vi "RDB Create Objects.vi"(8 "error in":errorcluster, 11 "Compiled.Settings":T5={"Name"="", "RDB Data Receive "=[], "RDB Data Sent"=[], "vclient"=path "", "Network Settings"={"IP adress"="127.0.0.1", "RDB"={"Protocol"=enum."UDP", "Tx Port"=48270, "Rx Port"=10, "Buffer Size"=204800, "Timeout"=10}, "SCP"={"Protocol"=enum."TCP", "Tx Port"=48191, "Rx Port"=48191, "Buffer Size"=204800, "Timeout"=10}}, "SensorInfos"=[], "mmanager"=path "", "Scenario Paths"=[], "Custom SCP Commands"=[]}) -> (0 "error out":errorcluster, 3 "RDB References":T1 {"RDB Send Reference"."RDB Data"."payload" format="%x"; "RDB Send Reference"."RDB Data"."timestamp" format="%<%.7X\n%x>T"; "RDB Send Reference"."RDB Data"."type" items=["FlexRay Data"=32, "FlexRay Null"=33, "FlexRay Symbol"=34, "Log Trigger"=225, "Start Trigger"=226]; "RDB Send Reference"."RDB Data"."cycle count" max=63 step=1; "RDB Receive Reference"."RDB Data"."payload" format="%x"; "RDB Receive Reference"."RDB Data"."timestamp" format="%<%.7X\n%x>T"; "RDB Receive Reference"."RDB Data"."type" items=["FlexRay Data"=32, "FlexRay Null"=33, "FlexRay Symbol"=34, "Log Trigger"=225, "Start Trigger"=226]; "RDB Receive Reference"."RDB Data"."cycle count" max=63 step=1})   [LabVIEW 2023, in "RDB.lvlib"]
uses:
  RDB.lvlib
  Shared/Compiled.Settings.ctl
  System Explorer/RDB Data.ctl
  RDB Object.ctl
  RDB Player Object.ctl
  Shared/Network Settings.ctl
  Shared/Protocol.ctl
  Shared/SensorInfos.ctl
  Shared/SensorInfo.ctl
  Shared/Sensor Name.ctl
  MM/MM Data.ctl
  MM/MM Objects.ctl
  MM/MM Object.ctl
  RDB References.ctl
  RDB Reference.ctl
  <vilib>/xnet/xnet.llb/XNET Frame FlexRay.ctl
  <vilib>/xnet/xnet.llb/XNET Frame Type FlexRay.ctl
  <vilib>/xnet/xnet.llb/XNET String To IO Name (Signal).vi
  <vilib>/xnet/xnet.llb/XNET Create Session (Conversion).vi
  <resource>/objmgr/xnet.rc
  Shared/Vires VTD Shared.lvlib
  MM/MM.lvlib
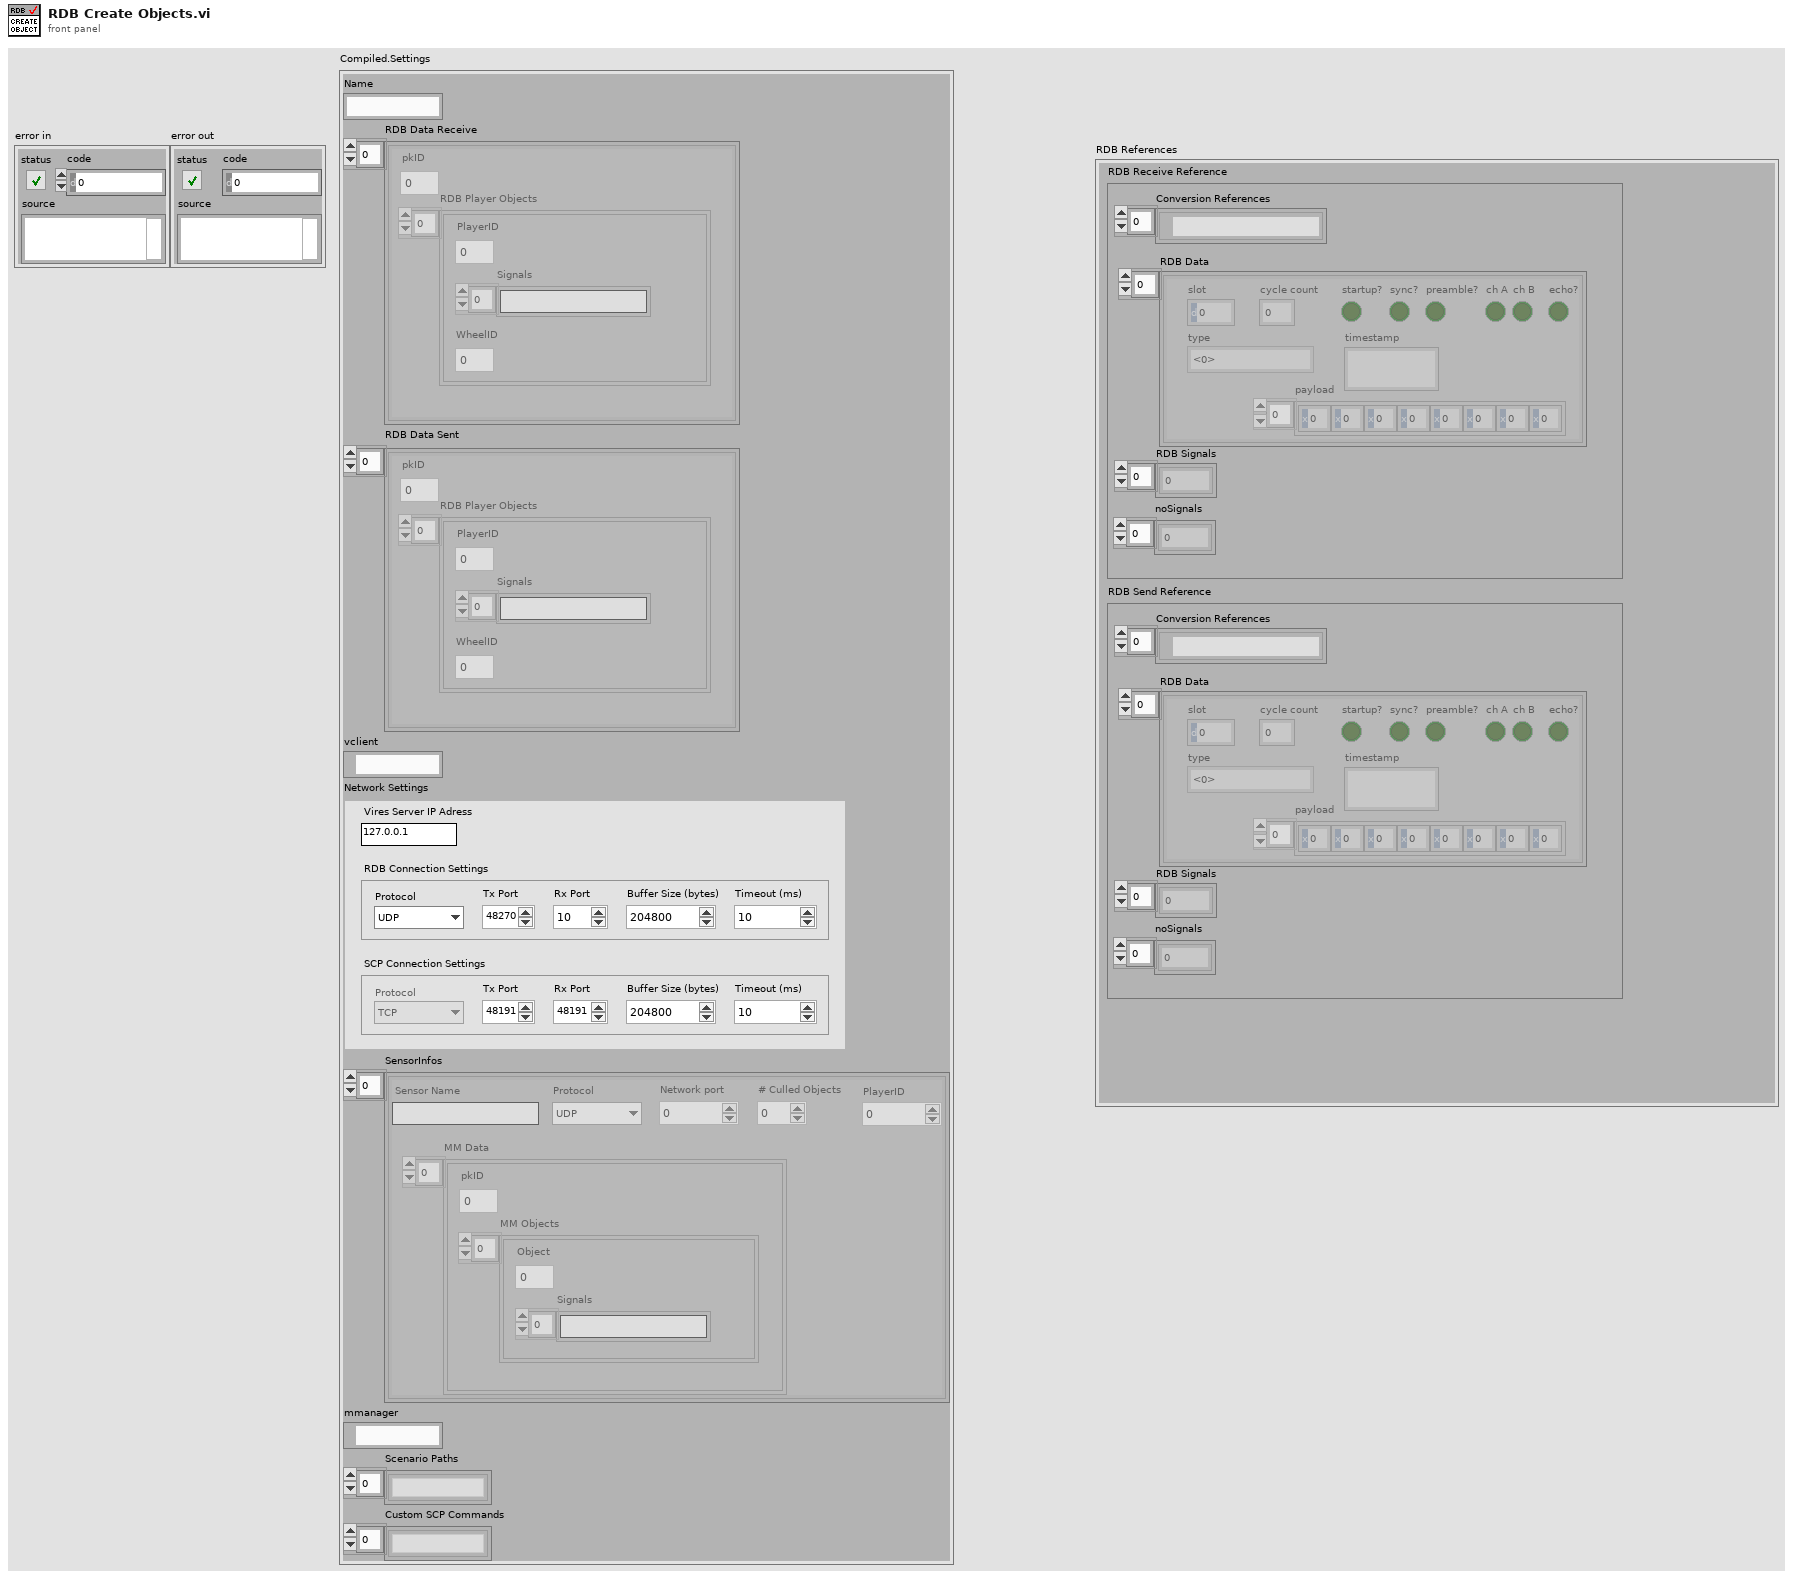
[diagram p1: front panel]
types:
  T1 = typedef "RDB.lvlib/RDB References.ctl" = cluster{"RDB Receive Reference":T2, "RDB Send Reference":T2}
  T2 = typedef "RDB.lvlib/RDB Reference.ctl" = cluster{"Conversion References":refnum<k21>[], "RDB Data":T3[], "RDB Signals":dbl[], "noSignals":i32[]}
  T3 = typedef "XNET Frame FlexRay.ctl" = cluster{"timestamp":timestamp, "payload":u8[], "slot":u16, "type":T4, "cycle count":u8, "startup?":bool, "sync?":bool, "preamble?":bool, "ch A":bool, "ch B":bool, "echo?":bool}
  T4 = typedef "XNET Frame Type FlexRay.ctl" = u8
  T5 = typedef "Vires VTD Shared.lvlib/Compiled.Settings.ctl" = cluster{"Name":string, "RDB Data Receive ":T6, "RDB Data Sent":T6, "vclient":path, "Network Settings":T9, "SensorInfos":T11, "mmanager":path, "Scenario Paths":string[], "Custom SCP Commands":string[]}
  T6 = typedef "Vires VTD Shared.lvlib/RDB Data.ctl" = T7[]
  T7 = typedef "RDB.lvlib/RDB Object.ctl" = cluster{"pkID":i32, "RDB Player Objects":T8[]}
  T8 = typedef "RDB.lvlib/RDB Player Object.ctl" = cluster{"PlayerID":i32, "Signals":string[], "WheelID":i32}
  T9 = typedef "Vires VTD Shared.lvlib/Network Settings.ctl" = cluster{"IP adress":string, "RDB":cluster{"Protocol":T10, "Tx Port":u16, "Rx Port":u16, "Buffer Size":i32, "Timeout":u16}, "SCP":cluster{"Protocol":T10, "Tx Port":u16, "Rx Port":u16, "Buffer Size":i32, "Timeout":u16}}
  T10 = typedef "Vires VTD Shared.lvlib/Protocol.ctl" = enum16{"UDP", "TCP"}
  T11 = typedef "Vires VTD Shared.lvlib/SensorInfos.ctl" = T12[]
  T12 = typedef "Vires VTD Shared.lvlib/SensorInfo.ctl" = cluster{"Sensor Name":T13, "Protocol":T10, "Network port":i32, "# Culled Objects":i32, "PlayerID":u8, "MM Data":T14}
  T13 = typedef "Vires VTD Shared.lvlib/Sensor Name.ctl" = string
  T14 = typedef "Vires VTD Shared.lvlib/MM Data.ctl" = T15[]
  T15 = typedef "MM.lvlib/MM Objects.ctl" = cluster{"pkID":i32, "MM Objects":T16[]}
  T16 = typedef "MM.lvlib/MM Object.ctl" = cluster{"Object":i32, "Signals":string[]}
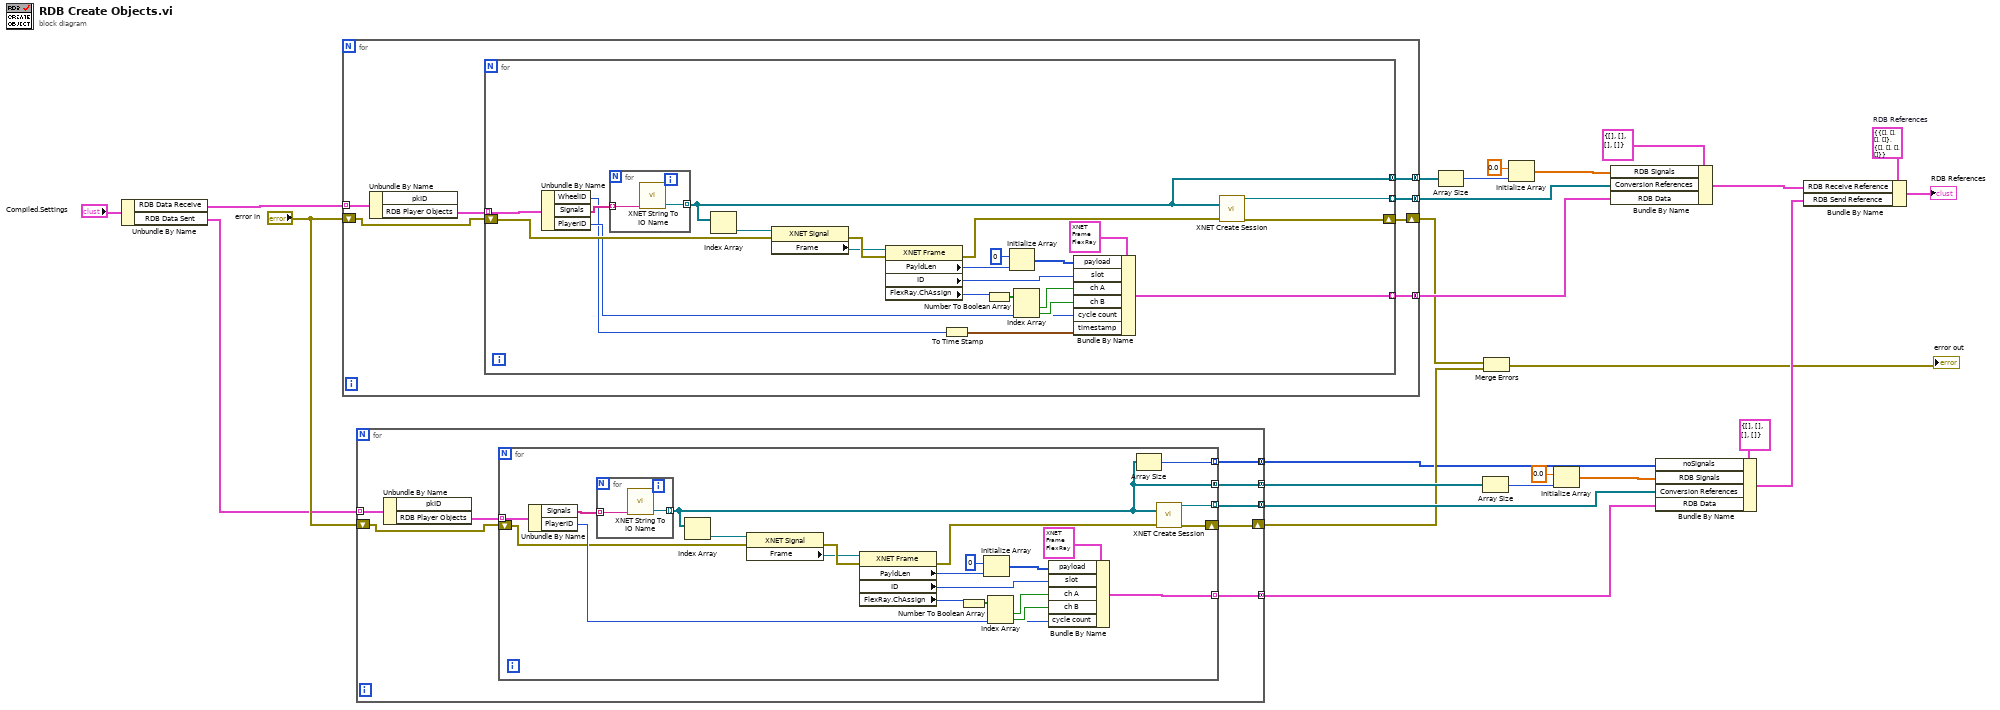
[diagram p0: block diagram]
diagram:
  w18 = T1 {"RDB Receive Reference"={"Conversion References"=[], "RDB Data"=[], "RDB Signals"=[], "noSignals"=[]}, "RDB Send Reference"={"Conversion References"=[], "RDB Data"=[], "RDB Signals"=[], "noSignals"=[]}}  # RDB References
  n1 = Unbundle By Name("Compiled.Settings") -> ("RDB Data Receive"=w7:T6, "RDB Data Sent"=w6:T6)
  n2 = for {
    tunnel: w7 -> [w33] mode=indexing
    shift-right: [w31] -> w3
    shift-left: "error in" -> [w30]
    tunnel: [w29] -> w22 mode=concatenating
    tunnel: [w27] -> w21 mode=concatenating
    tunnel: [w28] -> w20 mode=concatenating
    n3 = Unbundle By Name(w33) -> ("RDB Player Objects"=w32:T8[])  [unwired: 1 out]
    n4 = for {
      tunnel: w32 -> [w56] mode=indexing
      shift-right: [w55] -> w31
      shift-left: w30 -> [w54]
      tunnel: [w53] -> w29 mode=concatenating
      tunnel: [w38] -> w28 mode=indexing
      tunnel: [w34] -> w27 mode=indexing
      n5 = Unbundle By Name(w56) -> ("WheelID"=w36:i32, "Signals"=w51:string[], "PlayerID"=w39:i32)
      n6 = for {
        tunnel: w51 -> [w57] mode=indexing
        tunnel: [w58] -> w53 mode=indexing
        n7 = call-poly <vilib>:"XNET String To IO Name.vi"("string"=w57) -> ("XNET Signal"=w58:refnum<k21>)  [unwired: 4 out]
      }
      n8 = Index Array(array=w53) -> (element=w40:refnum<k21>)  [unwired: 1 in]
      n9 = property class="XNET Signal"(reference=w40, error in=w54) -> (error out=w50:errorcluster, "Frame"=w49:refnum<k21>)  [unwired: 1 out]
      n10 = property class="XNET Frame"(reference=w49, error in=w50) -> (error out=w52:errorcluster, "PayldLen"=w42:u32, "ID"=w44:u32, "FlexRay.ChAssign"=w45:u32)  [unwired: 1 out]
      n11 = To Time Stamp(1:w36) -> (0:w35:timestamp)
      n12 = Number To Boolean Array(number=w45) -> (Boolean array=w41:bool[])
      n13 = Initialize Array(0 ("element"), w42) -> (w43:i32[])
      n14 = Index Array(array=w41) -> (element #1=w46:bool, element #2=w47:bool)  [unwired: 2 in]
      n15 = Bundle By Name(cluster=T3 {"timestamp"=timestamp(0 s since 1904-01-01), "payload"=[], "slot"=1, "type"=32, "cycle count"=0, "startup?"=FALSE, "sync?"=FALSE, "preamble?"=FALSE, "ch A"=FALSE, "ch B"=FALSE, "echo?"=FALSE} ("FlexRay frame"), "payload"=w43, "slot"=w44, "ch A"=w46, "ch B"=w47, "cycle count"=w39, "timestamp"=w35) -> (w38:T3)
      n16 = call-poly <vilib>:"XNET Create Session.vi"("signal list"=w53, "error in (no error)"=w52) -> ("session out"=w34:refnum<k21>, "error out"=w55:errorcluster)  [unwired: 12 in]
    }
  }
  n17 = for {
    tunnel: w6 -> [w66] mode=indexing
    shift-right: [w64] -> w2
    shift-left: "error in" -> [w63]
    tunnel: [w62] -> w12 mode=concatenating
    tunnel: [w61] -> w13 mode=concatenating
    tunnel: [w60] -> w14 mode=concatenating
    tunnel: [w59] -> w1 mode=concatenating
    n18 = Unbundle By Name(w66) -> ("RDB Player Objects"=w65:T8[])  [unwired: 1 out]
    n19 = for {
      tunnel: w65 -> [w88] mode=indexing
      tunnel: [w73] -> w60 mode=indexing
      tunnel: [w69] -> w61 mode=indexing
      shift-right: [w71] -> w64
      shift-left: w63 -> [w70]
      tunnel: [w68] -> w62 mode=concatenating
      tunnel: [w67] -> w59 mode=indexing
      n20 = Unbundle By Name(w88) -> ("Signals"=w87:string[], "PlayerID"=w74:i32)
      n21 = for {
        tunnel: w87 -> [w90] mode=indexing
        tunnel: [w89] -> w68 mode=indexing
        n22 = call-poly <vilib>:"XNET String To IO Name.vi"("string"=w90) -> ("XNET Signal"=w89:refnum<k21>)  [unwired: 4 out]
      }
      n23 = Index Array(array=w68) -> (element=w75:refnum<k21>)  [unwired: 1 in]
      n24 = property class="XNET Signal"(reference=w75, error in=w70) -> (error out=w86:errorcluster, "Frame"=w85:refnum<k21>)  [unwired: 1 out]
      n25 = property class="XNET Frame"(reference=w85, error in=w86) -> (error out=w72:errorcluster, "PayldLen"=w78:u32, "ID"=w80:u32, "FlexRay.ChAssign"=w81:u32)  [unwired: 1 out]
      n26 = Number To Boolean Array(number=w81) -> (Boolean array=w76:bool[])
      n27 = Initialize Array(u8 0 ("element"), w78) -> (w79:u8[])
      n28 = Index Array(array=w76) -> (element #1=w82:bool, element #2=w83:bool)  [unwired: 2 in]
      n29 = Bundle By Name(cluster=T3 {"timestamp"=timestamp(0 s since 1904-01-01), "payload"=[], "slot"=1, "type"=32, "cycle count"=0, "startup?"=FALSE, "sync?"=FALSE, "preamble?"=FALSE, "ch A"=FALSE, "ch B"=FALSE, "echo?"=FALSE} ("FlexRay frame"), "payload"=w79, "slot"=w80, "ch A"=w82, "ch B"=w83, "cycle count"=w74) -> (w73:T3)
      n30 = Array Size(array=w68) -> (size(s)=w67:i32)
      n31 = call-poly <vilib>:"XNET Create Session.vi"("signal list"=w68, "error in (no error)"=w72) -> ("session out"=w69:refnum<k21>, "error out"=w71:errorcluster)  [unwired: 12 in]
    }
  }
  n32 = Array Size(array=w22) -> (size(s)=w23:i32)
  n33 = Array Size(array=w12) -> (size(s)=w11:i32)
  n34 = Merge Errors(w3, w2) -> (→"error out":errorcluster)
  n35 = Initialize Array(0.0 ("element"), w23) -> (w24:dbl[])
  n36 = Initialize Array(0.0 ("element"), w11) -> (w10:dbl[])
  n37 = Bundle By Name(cluster=T2 {"Conversion References"=[], "RDB Data"=[], "RDB Signals"=[], "noSignals"=[]} ("RDB Reference"), "RDB Signals"=w24, "Conversion References"=w21, "RDB Data"=w20) -> (w17:T2)
  n38 = Bundle By Name(cluster=T2 {"Conversion References"=[], "RDB Data"=[], "RDB Signals"=[], "noSignals"=[]} ("RDB Reference"), "noSignals"=w1, "RDB Signals"=w10, "Conversion References"=w13, "RDB Data"=w14) -> (w5:T2)
  n39 = Bundle By Name(cluster=w18, "RDB Receive Reference"=w17, "RDB Send Reference"=w5) -> (→"RDB References":T1)
